vi "test_Path (relative).vi"(8 "error in (no error)":errorcluster, 11 "TestCase in":refnum<class "Test Read File.lvclass">) -> (0 "error out":errorcluster, 3 "TestCase out":refnum<class "Test Read File.lvclass">)   [LabVIEW 2019, in "Test Read File.lvclass"]
uses:
  Test Read File.lvclass
  C:/Program Files/National Instruments/LabVIEW 2024/vi.lib/Astemes/LUnit/Test Case.lvclass
  Test Read File.lvclass/Test Read File.ctl
  <vilib>/Astemes/LUnit/Test Case.lvclass/Test Case.ctl
  e5bb9074-a9a1-47e8-b80f-714184f69ea6.vi
  <vilib>/Astemes/LUnit/Core/LUnit Test Case/Private/Append Pass Result.vi
  <vilib>/Astemes/LUnit/Core/LUnit Test Case/Private/Append Fail Result.vi
  e5bb9074-a9a1-47e8-b80f-714184f69ea6.vi/9c5d11cd-9439-4240-a1ee-d9baace9c924.vi
  <vilib>/Astemes/LUnit/Core/LUnit Test Case/Private/Run In UI.vi
  <vilib>/Utility/error.llb/Clear Errors.vi
  Read/Read Section - Path.vi
  TSC File IO.lvlib
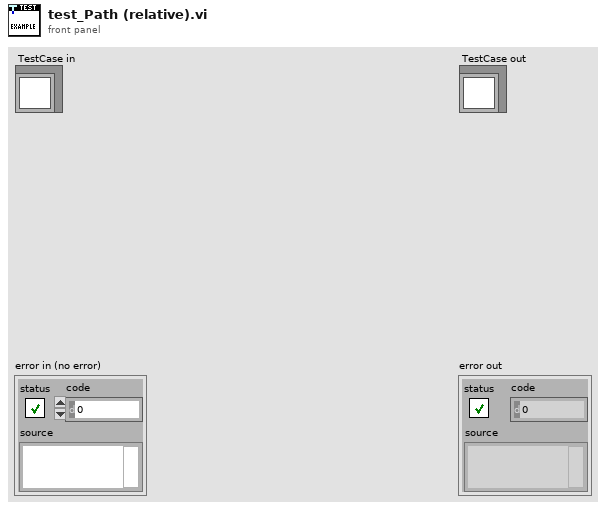
[diagram p1: front panel]
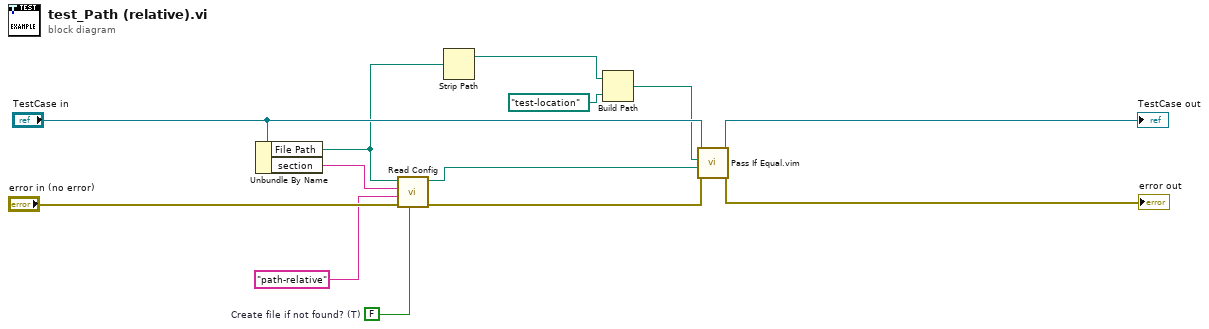
[diagram p0: block diagram]
diagram:
  w8 = FALSE  # Create file if not found? (T)
  n1 = Unbundle By Name("TestCase in") -> ("File Path"=w2:path, "section"=w1:string)
  n2 = call-poly "Read Config.vi"("Create file if not found? (T)"=w8, "error in (no error)"="error in (no error)", "key"="path-relative", "section"=w1, "Path"=w2) -> ("error out"=w7:errorcluster, "value"=w6:path)  [unwired: 5 in]
  n3 = Strip Path(path=w2) -> (stripped path=w4:path)  [unwired: 1 out]
  n4 = Build Path(base path=w4, name or relative path=path "test-location") -> (appended path=w3:path)
  n5 = call "Pass If Equal.vim"("error in (no error)"=w7, "Actual"=w6, "Expected"=w3, "LUnit Test Case In"="TestCase in") -> ("error out"=→"error out":errorcluster, "LUnit Test Case Out"=→"TestCase out":refnum<class "Test Read File.lvclass">)  [unwired: 6 in]
